vi "generate_heap_and_hill_coordinates_3.vi"(8 "error in (no error)":errorcluster, 10 "ants":refnum<class "ant_base.lvclass">[](array[class])) -> (0 "error out":errorcluster, 1 "hillsArray":T5[](array[typedef]), 2 "foodHeapsArray":T1[](array[typedef])=[{"centerCoordinates"={"X"=100, "Y"=100}, "radius"=20.0, "volume"=1000, "Color"=5876991}, {"centerCoordinates"={"X"=140, "Y"=240}, "radius"=10.0, "volume"=10, "Color"=0}])   [LabVIEW 2015, in "world.lvlib" / "world.lvclass"]
doc: "generate coordinates of hills and heaps\nCreated by Artem Shevelev\nshevelev.pro\nartem@shevelev.pro\nLabVIEW Portal: https://labviewportal.org/memberlist.php?mode=viewprofile&u=2340"
uses:
  world.lvclass
  typedefs/worldPoint.ctl
  world.lvlib
  typedefs/worldPoint_cluster.ctl
  typedefs/anthill_cluster.ctl
  ant_base/ant_base.lvclass
  typedefs/amountOfFood.ctl
  typedefs/foodHeap_cluster.ctl
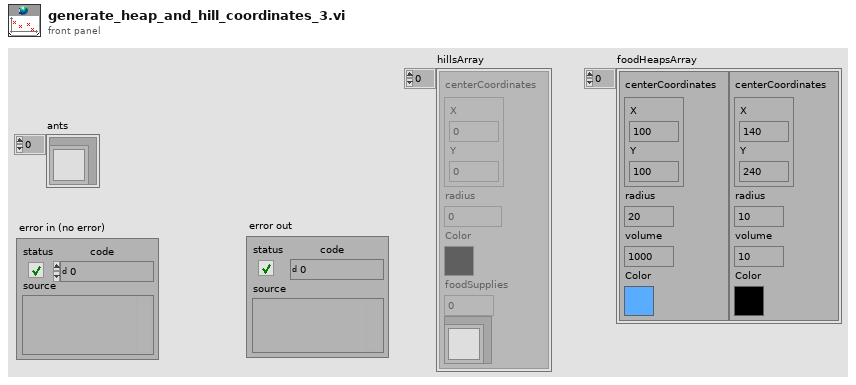
[diagram p1: front panel]
types:
  T1 = typedef "world.lvlib/foodHeap_cluster.ctl" = cluster{"centerCoordinates":T2, "radius":dbl, "volume":T4, "Color":u32}
  T2 = typedef "world.lvlib/worldPoint_cluster.ctl" = cluster{"X":T3, "Y":T3}
  T3 = typedef "world.lvlib/worldPoint.ctl" = i16
  T4 = typedef "world.lvlib/amountOfFood.ctl" = i32
  T5 = typedef "world.lvlib/anthill_cluster.ctl" = cluster{"centerCoordinates":T2, "radius":dbl, "Color":u32, "foodSupplies":T4, "antType":refnum<class "ant_base.lvclass">}
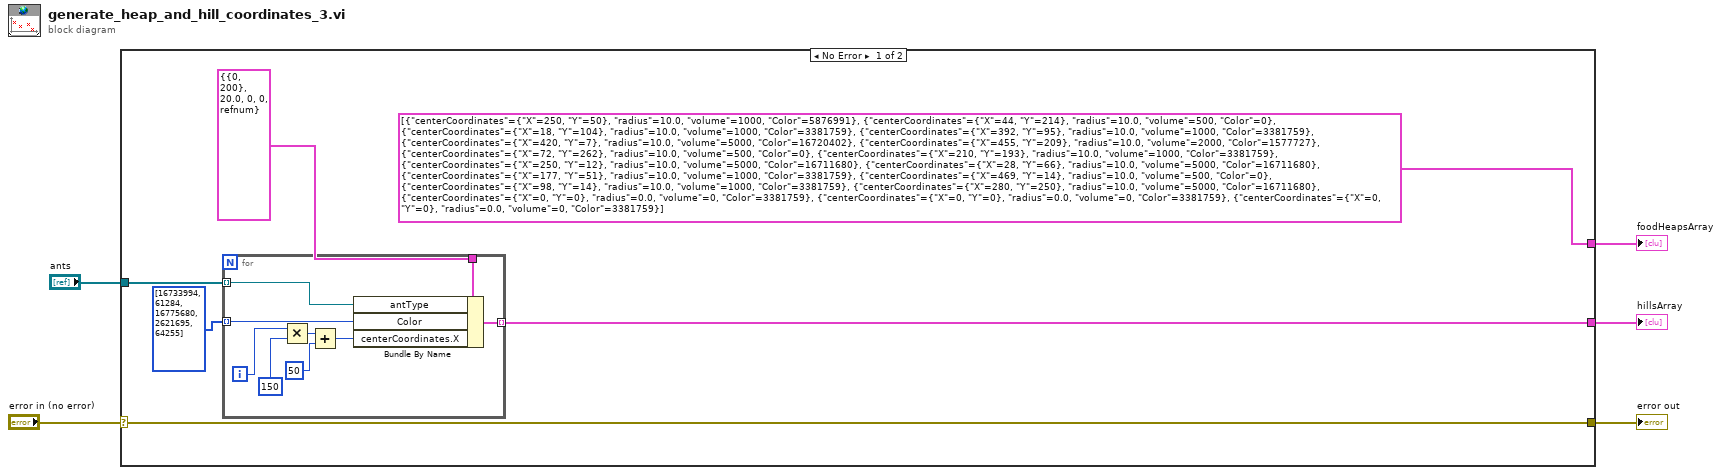
[diagram p0: block diagram]
diagram:
  n1 = case shown="No Error" "error in (no error)" {
    selector: "error in (no error)" -> [w8 w21]
    tunnel: [w9 _] -> w5
    tunnel: [T1[] [{"centerCoordinates"={"X"=250, "Y"=50}, "radius"=10.0, "volume"=1000, "Color"=5876991}, {"centerCoordinates"={"X"=44, "Y"=214}, "radius"=10.0, "volume"=500, "Color"=0}, {"centerCoordinates"={"X"=18, "Y"=104}, "radius"=10.0, "volume"=1000, "Color"=3381759}, {"centerCoordinates"={"X"=392, "Y"=95}, "radius"=10.0, "volume"=1000, "Color"=3381759}, {"centerCoordinates"={"X"=420, "Y"=7}, "radius"=10.0, "volume"=5000, "Color"=16720402}, {"centerCoordinates"={"X"=455, "Y"=209}, "radius"=10.0, "volume"=2000, "Color"=1577727}, {"centerCoordinates"={"X"=72, "Y"=262}, "radius"=10.0, "volume"=500, "Color"=0}, {"centerCoordinates"={"X"=210, "Y"=193}, "radius"=10.0, "volume"=1000, "Color"=3381759}, {"centerCoordinates"={"X"=250, "Y"=12}, "radius"=10.0, "volume"=5000, "Color"=16711680}, {"centerCoordinates"={"X"=28, "Y"=66}, "radius"=10.0, "volume"=5000, "Color"=16711680}, {"centerCoordinates"={"X"=177, "Y"=51}, "radius"=10.0, "volume"=1000, "Color"=3381759}, {"centerCoordinates"={"X"=469, "Y"=14}, "radius"=10.0, "volume"=500, "Color"=0}, {"centerCoordinates"={"X"=98, "Y"=14}, "radius"=10.0, "volume"=1000, "Color"=3381759}, {"centerCoordinates"={"X"=280, "Y"=250}, "radius"=10.0, "volume"=5000, "Color"=16711680}, {"centerCoordinates"={"X"=0, "Y"=0}, "radius"=0.0, "volume"=0, "Color"=3381759}, {"centerCoordinates"={"X"=0, "Y"=0}, "radius"=0.0, "volume"=0, "Color"=3381759}, {"centerCoordinates"={"X"=0, "Y"=0}, "radius"=0.0, "volume"=0, "Color"=3381759}] ("foodHeapsArray") _] -> w4
    tunnel: [w8 w21] -> w2
    tunnel: "ants" -> [w7 _]
    frame No Error {
      n2 = for {
        tunnel: T5 {"centerCoordinates"={"X"=0, "Y"=200}, "radius"=20.0, "Color"=0, "foodSupplies"=0, "antType"=refnum} ("anthill") -> [w20]
        tunnel: u32[] [16733994, 61284, 16775680, 2621695, 64255] ("Color") -> [w19] mode=indexing
        tunnel: [w16] -> w9 mode=indexing
        tunnel: w7 -> [w15] mode=indexing
        i -> [w13]
        n3 = Multiply(x=w13, y=150) -> (x*y=w18:i32)
        n4 = Add(x=w18, y=50) -> (x+y=w14:i32)
        n5 = Bundle By Name(cluster=w20, "antType"=w15, "Color"=w19, "centerCoordinates.X"=w14) -> (w16:T5)
      }
    }
    frame Error {
    }
  }
  "error out" <- w2
  "hillsArray" <- w5
  "foodHeapsArray" <- w4
